vi "Exercise 5-2.vi"() -> ()   [LabVIEW 2014]
panel:
  out "Small Cluster":cluster{"Boolean 1":bool, "Slide Value":dbl} {"Slide Value" format="%.2g"}
  out "Boolean 2":bool
  out "Numeric":dbl format="%.2g"
  in  "stop":bool
  out "Modified Cluster":T1 {"Slide" scale=0.0..10.0; "Numeric" format="%.2f"}
  in  "Cluster":T1 {"Slide" scale=0.0..10.0; "Numeric" format="%.2f"}
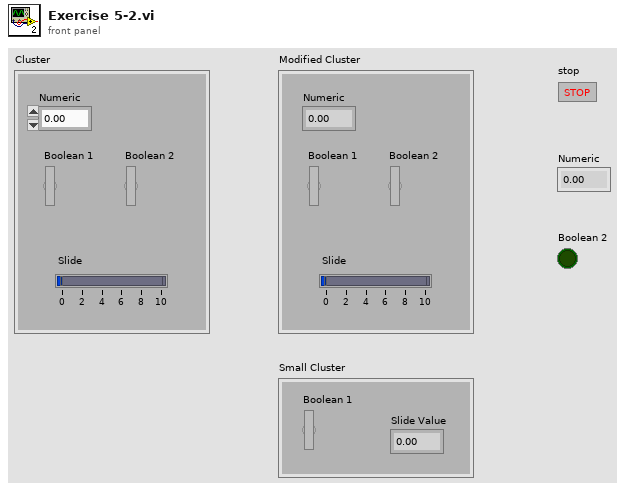
[diagram p1: front panel]
types:
  T1 = cluster{"Numeric":dbl, "Boolean 1":bool, "Boolean 2":bool, "Slide":dbl}
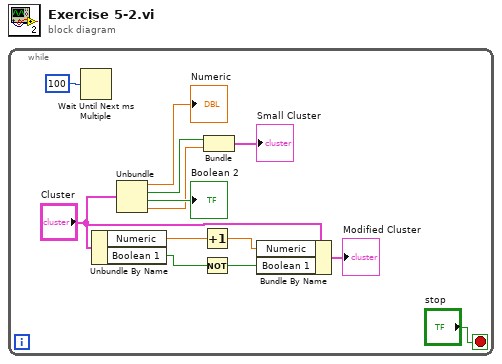
[diagram p0: block diagram]
diagram:
  n1 = while {
    stop <- "stop" stop-if-true
    n2 = Wait Until Next ms Multiple(millisecond multiple=100) -> ()  [unwired: 1 out]
    n3 = Unbundle By Name("Cluster") -> ("Numeric"=w12:dbl, "Boolean 1"=w11:bool)
    n4 = Unbundle("Cluster") -> ("Numeric"=→"Numeric":dbl, "Boolean 1"=w5:bool, "Boolean 2"=→"Boolean 2":bool, "Slide"=w4:dbl)
    n5 = Increment(x=w12) -> (x+1=w9:dbl)
    n6 = Not(x=w11) -> (.not. x?=w8:bool)
    n7 = Bundle("Boolean 1"=w5, "Slide"=w4) -> (→"Small Cluster":cluster{"Boolean 1":bool, "Slide":dbl})  [unwired: 1 in]
    n8 = Bundle By Name(cluster="Cluster", "Numeric"=w9, "Boolean 1"=w8) -> (→"Modified Cluster":T1)
  }
